vi "图像处理.vi"() -> ()   [LabVIEW 2023]
uses:
  <vilib>/vision/NI_Vision_Development_Module.lvlib
panel:
  out "Area":dbl
  out "错误输出 2":errorcluster caption="错误输出"
  in  "停止":bool
  in  "Center of Mass 2":cluster{"X":dbl, "Y":dbl}
  in  "数值":i32
  out "Threshold Image":T1(plugin-control)
  out "Selected Particle Report":T2 {"Orientation" format="%.2f"; "Center of Mass"."Y" format="%.2f"; "Center of Mass"."X" format="%.2f"}
  out "Center of Mass":cluster{"X":dbl, "Y":dbl}
  in  "获取种子图像":bool
  in  "File Path":path
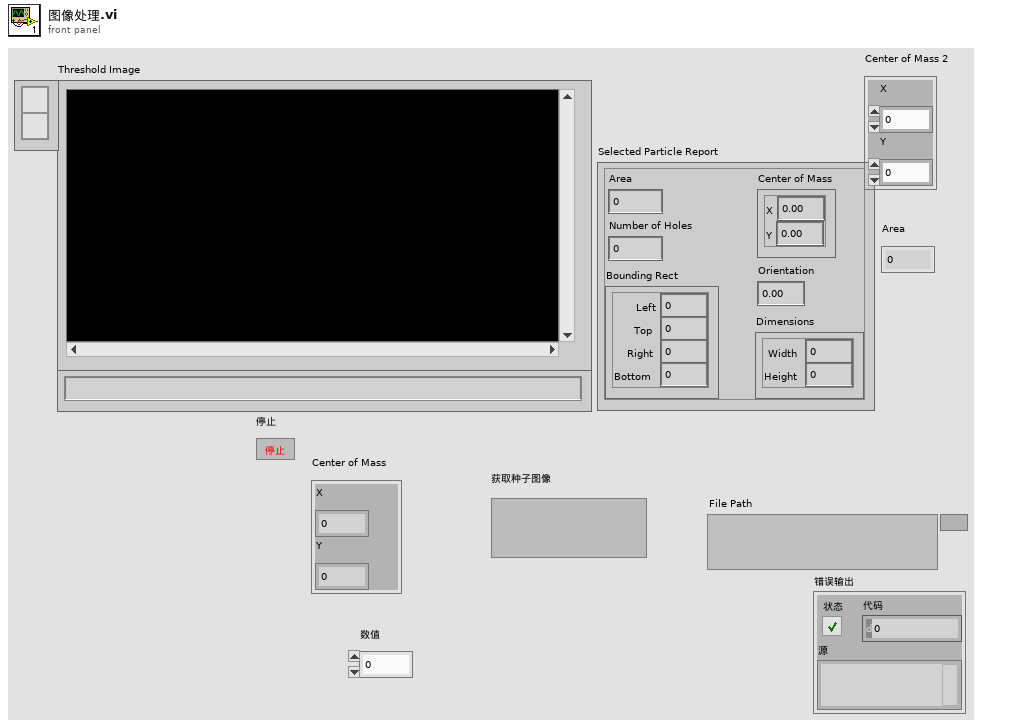
[diagram p1: front panel]
types:
  T1 = typedef "IMAQ Image.ctl" = refnum<image>
  T2 = cluster{"Area":dbl, "Number of Holes":dbl, "Bounding Rect":cluster{"Left":dbl, "Top":dbl, "Right":dbl, "Bottom":dbl}, "Center of Mass":cluster{"X":dbl, "Y":dbl}, "Orientation":dbl, "Dimensions":cluster{"Width":dbl, "Height":dbl}}
  T3 = typedef "控件 1.ctl" = enum16{"等待用户输入", "获取种子图像", "分析破损种子坐标"}
  T4 = cluster{"Area":dbl, "Number of Holes":dbl, "Bounding Rect":cluster{"Left":dbl, "Top":dbl, "Right":dbl, "Bottom":dbl}, "Center of Mass":cluster{"X":dbl, "Y":dbl}, "Orientation":dbl, "Dimensions":cluster{"Width":dbl, "Height":dbl}}[]
  T5 = cluster{"Left":dbl, "Top":dbl, "Right":dbl, "Bottom":dbl}
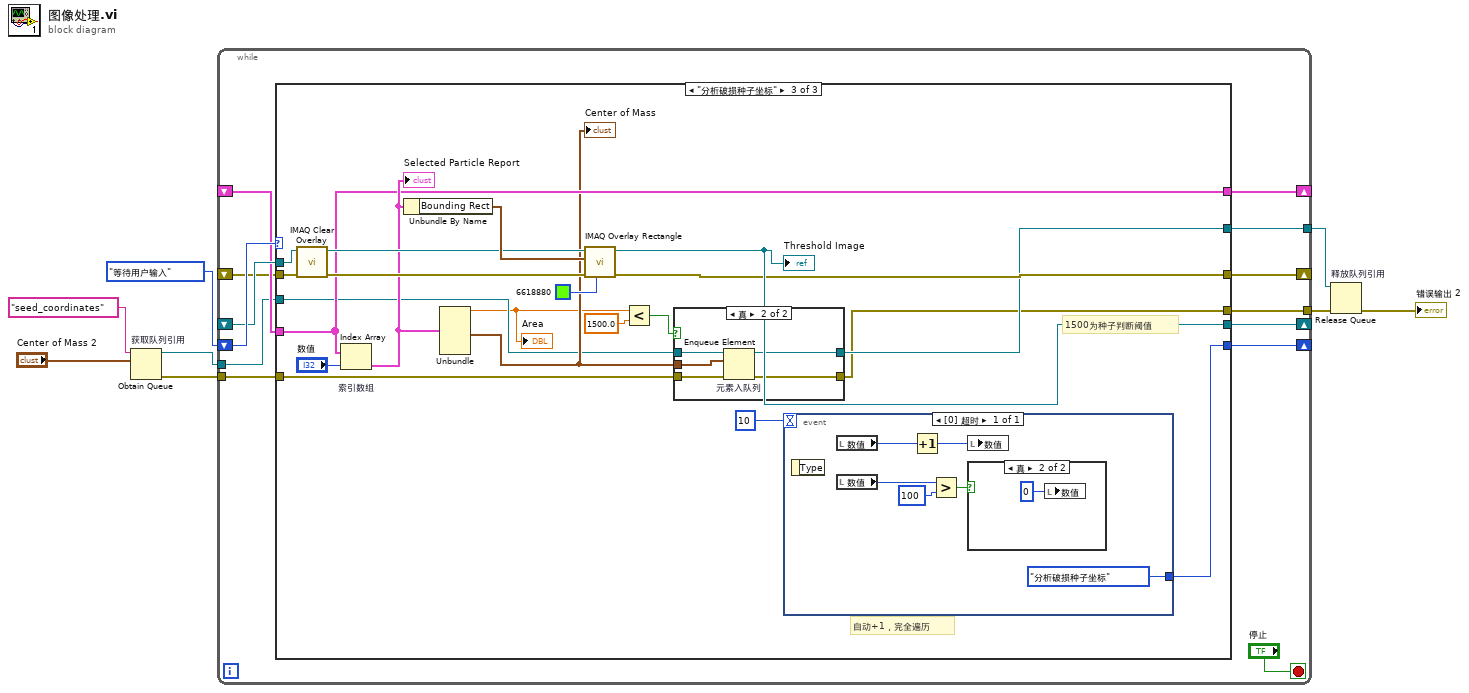
[diagram p0: block diagram]
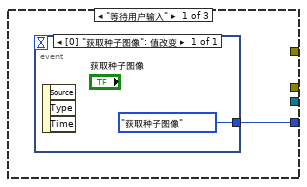
[diagram p2: hidden frame]
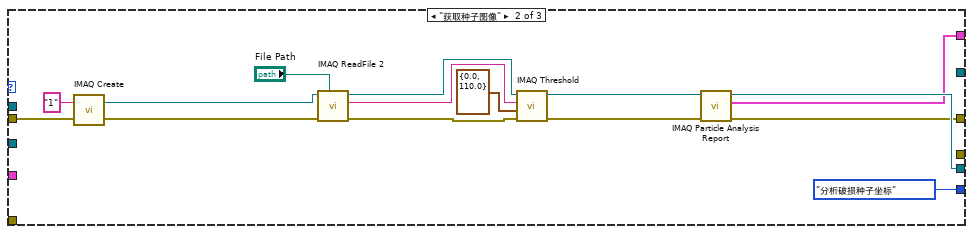
[diagram p3: hidden frame]
diagram:
  n1 = Obtain Queue "获取队列引用"(name (unnamed)="seed_coordinates" ("名称（未命名）"), element data type="Center of Mass 2") -> (queue out=w5:refnum<queue>, error out=w6:errorcluster)  [unwired: 3 in, 1 out]
  n2 = while {
    shift-right: [w20] -> _
    shift-left: 控件_1."等待用户输入" ("枚举") -> [w21]
    shift-right: [w19] -> _
    shift-left: _ -> [w16]
    shift-right: [w18] -> _
    shift-left: _ -> [w14]
    shift-right: [w17] -> _
    shift-left: _ -> [w15]
    tunnel: w5 -> [w13]
    tunnel: w6 -> [w12]
    tunnel: [w10] -> w3
    tunnel: [w9] -> w2
    stop <- "停止" stop-if-true
    n3 = case shown="\"分析破损种子坐标\"" w21 {
      tunnel: [w22 控件_1."分析破损种子坐标" ("枚举") w47] -> w20
      tunnel: [_ w29 w57] -> w19
      tunnel: [_ w28 w56] -> w18
      tunnel: [_ w27 w49] -> w17
      tunnel: w16 -> [_ _ w59]
      tunnel: w15 -> [_ _ w49]
      tunnel: w14 -> [_ w26 w58]
      tunnel: w13 -> [_ _ w43]
      tunnel: w12 -> [_ _ w42]
      tunnel: [_ _ w41] -> w10
      tunnel: [_ _ w40] -> w9
      frame "等待用户输入" {
        n4 = event shown="[0] \"获取种子图像\": 值改变" {
          selector: _ -> [_]
          dyn-events: _ -> [_]
          timeout: _ -> [_]
          tunnel: [控件_1."获取种子图像" ("枚举")] -> w22
          event "获取种子图像": Value Change {
            n5 = event-data() -> ()  [unwired: 1 in, 3 out]
          }
        }
      }
      frame "获取种子图像" {
        n6 = call "IMAQ Create"("Image Name"="1", "error in (no error)"=w26) -> ("New Image"=w37:T1, "error out"=w36:errorcluster)  [unwired: 3 in]
        n7 = call "IMAQ ReadFile 2"("File Path"="File Path", "error in (no error)"=w36, "Image"=w37) -> ("error out"=w34:errorcluster, "File Type out"=w25:string, "Image Out"=w35:T1)  [unwired: 4 in, 2 out]
        n8 = call "IMAQ Threshold"("error in (no error)"=w34, "Range"=cluster{"Lower value":sgl, "Upper value":sgl} {"Lower value"=0.0, "Upper value"=110.0}, "Image Dst"=w25, "Image Src"=w35) -> ("error out"=w33:errorcluster, "Image Dst Out"=w32:T1)  [unwired: 6 in]
        n9 = call "IMAQ Particle Analysis Report"("error in (no error)"=w33, "Image"=w32) -> ("error out"=w28:errorcluster, "Particle Reports (Pixels)"=w27:T4, "Image Out (duplicate)"=w29:T1)  [unwired: 4 in, 3 out]
      }
      frame "分析破损种子坐标" {
        # "1500为种子判断阈值"
        # "自动+1，完全遍历"
        n10 = call "IMAQ Clear Overlay"("error in (no error)"=w58, "Image"=w59) -> ("error out"=w52:errorcluster, "Image Out"=w53:T1)  [unwired: 8 in]
        n11 = Index Array "索引数组"(array=w49, index="数值") -> (element=w51:T2)
        "Selected Particle Report" <- w51
        n12 = Unbundle By Name(w51) -> ("Bounding Rect"=w55:T5)
        n13 = Unbundle(w51) -> ("Area"=w39:dbl, "Center of Mass"=w45:cluster{"X":dbl, "Y":dbl})  [unwired: 4 out]
        "Center of Mass" <- w45
        "Area" <- w39
        n14 = call "IMAQ Overlay Rectangle"("Color"=u32 6618880, "error in (no error)"=w52, "Rectangle"=w55, "Image"=w53) -> ("error out"=w56:errorcluster, "Image Out"=w57:T1)  [unwired: 6 in]
        "Threshold Image" <- w57
        n15 = Less?(x=w39, y=1500.0) -> (x < y?=w44:bool)
        n16 = case shown="真" w44 {
          tunnel: w45 -> [_ w64]
          tunnel: [_ w63] -> w41
          tunnel: w43 -> [_ w62]
          tunnel: [_ w61] -> w40
          tunnel: w42 -> [_ w60]
          frame False {
          }
          frame True {
            n17 = Enqueue Element "元素入队列"(queue=w62, element=w64, error in (no error)=w60) -> (queue out=w63:refnum<queue>, error out=w61:errorcluster)  [unwired: 1 in, 1 out]
          }
        }
        n18 = event shown="[0] 超时" {
          selector: _ -> [_]
          dyn-events: _ -> [_]
          timeout: 10 -> [_]
          tunnel: [控件_1."分析破损种子坐标" ("枚举")] -> w47
          event Timeout {
            n19 = event-data() -> ()  [unwired: 1 in, 1 out]
            n20 = local read "数值"() -> (w69:i32)
            n21 = local read "数值"() -> (w67:i32)
            n22 = Increment(x=w69) -> (x+1=w70:i32)
            n23 = Greater?(x=w67, y=100) -> (0:w68:bool)
            n24 = local write "数值"(w70) -> ()
            n25 = case shown="真" w68 {
              frame False {
              }
              frame True {
                n26 = local write "数值"(0 ("y")) -> ()
              }
            }
          }
        }
      }
    }
  }
  n27 = Release Queue "释放队列引用"(queue=w3, error in (no error)=w2) -> (error out=→"错误输出 2":errorcluster)  [unwired: 1 in, 2 out]
